vi "Get and Set Focus Key.vi"(8 "错误输入（无错误）":errorcluster, 9 "Mode":enum16{"Read", "Write"}(ring), 10 "FocusKey In":T1 caption="Focuskey In", 11 "Ctl Ref In":refnum<vi>) -> (0 "错误输出":errorcluster, 2 "FocusKey Out":T1, 3 "Ctl Ref Out":refnum<vi>)   [LabVIEW 2012, in "CtrlRef.lvlib"]
uses:
  CtrlRef.lvlib
  <vilib>/Utility/miscctls.llb/LVKeyNavTypeDef.ctl
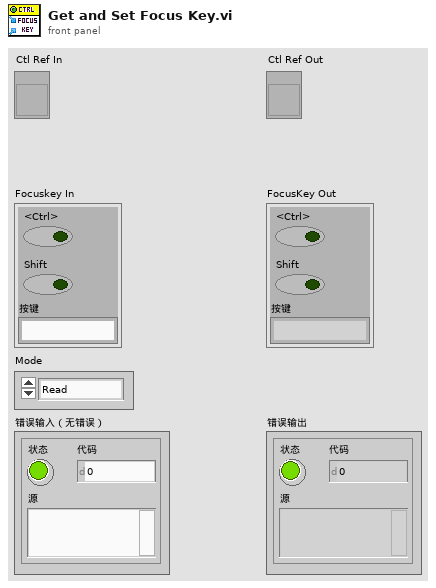
[diagram p1: front panel]
types:
  T1 = typedef "LVKeyNavTypeDef.ctl" = cluster{"Control":bool, "Shift":bool, "Key":string}
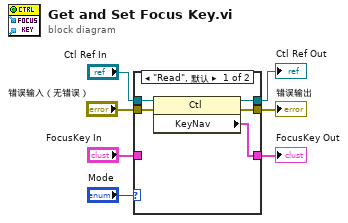
[diagram p0: block diagram]
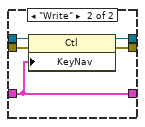
[diagram p2: hidden frame]
diagram:
  n1 = case shown="\"Read\", 默认" "Mode" {
    tunnel: "Ctl Ref In" -> [w12 w16]
    tunnel: "错误输入（无错误）" -> [w11 w17]
    tunnel: [w10 w14] -> w5
    tunnel: [w9 w15] -> w4
    tunnel: [w8 w13] -> w2
    tunnel: "FocusKey In" -> [_ w13]
    frame "Read", Default {
      n2 = property class="Ctl"(reference=w12, error in=w11) -> (reference out=w9:refnum<vi>, error out=w10:errorcluster, "KeyNav"=w8:T1)
    }
    frame "Write" {
      n3 = property class="Ctl"(reference=w16, error in=w17, "KeyNav"=w13) -> (reference out=w15:refnum<vi>, error out=w14:errorcluster)
    }
  }
  "错误输出" <- w5
  "Ctl Ref Out" <- w4
  "FocusKey Out" <- w2
